vi "Integrator.vi"() -> ()   [LabVIEW 2019]
panel:
  out "Original Wave":dbl[](graph)=[0.0, 0.6180339887498948, 1.1755705045849463, 1.6180339887498947, 1.902113032590307, 2.0, 1.9021130325903073, 1.618033988749895, 1.1755705045849465, 0.6180339887498959, 2.4492935982947064e-16, -0.6180339887498946, -1.1755705045849454, -1.6180339887498936, -1.902113032590307, -2.0, -1.9021130325903073, -1.6180339887498962, -1.175570504584948, -0.6180339887498953, -4.898587196589413e-16, 0.6180339887498927, 1.1755705045849458, 1.6180339887498936, 1.9021130325903064, 2.0, 1.9021130325903084, 1.6180339887498951, 1.1755705045849467, 0.6180339887498989, 7.347880794884119e-16, -0.6180339887498908, -1.1755705045849456, -1.6180339887498945, -1.9021130325903057, -2.0, -1.9021130325903086, -1.6180339887498953, -1.175570504584947, -0.6180339887498991]
  in  "Amplitude":dbl=2.0
  out "Integrated Wave":dbl[](graph)=[0.0, 6.180339887498948e-05, 0.0001793604493334841, 0.0003411638482084736, 0.0005313751514675043, 0.0007313751514675043, 0.000921586454726535, 0.0010833898536015245, 0.0012009469040600192, 0.0012627503029350087, 0.0012627503029350087, 0.0012009469040600192, 0.0010833898536015247, 0.0009215864547265354, 0.0007313751514675046, 0.0005313751514675046, 0.00034116384820847385, 0.00017936044933348423, 6.180339887498941e-05, -1.2197274440461925e-19, -1.7095861637051338e-19, 6.18033988749891e-05, 0.0001793604493334837, 0.0003411638482084731, 0.0005313751514675037, 0.0007313751514675037, 0.0009215864547265346, 0.001083389853601524, 0.0012009469040600187, 0.0012627503029350087, 0.0012627503029350087, 0.0012009469040600196, 0.001083389853601525, 0.0009215864547265357, 0.0007313751514675051, 0.0005313751514675052, 0.0003411638482084743, 0.00017936044933348474, 6.180339887499005e-05, 1.3552527156068805e-19]
  out "Integration Sum":dbl=1.3552527156068805e-19
  out "No. of\nsamples":dbl=40.0
  in  "No. of\ncycles":dbl=2.0
  in  "fs":dbl=10000.0
  in  "Phase":dbl
  in  "f":dbl=500.0
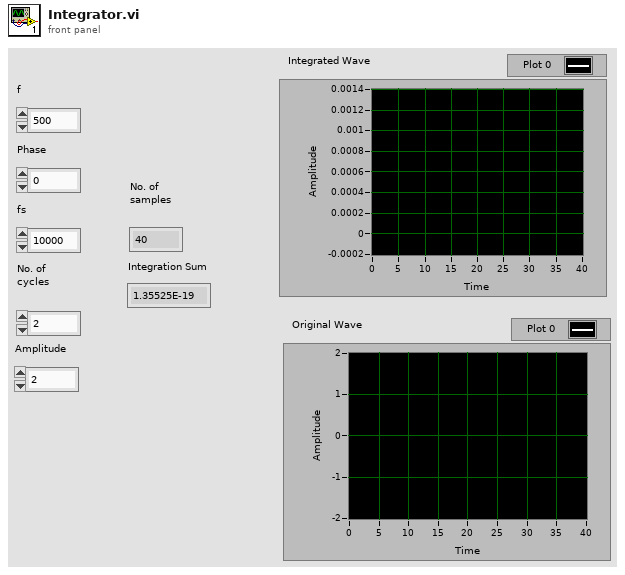
[diagram p1: front panel]
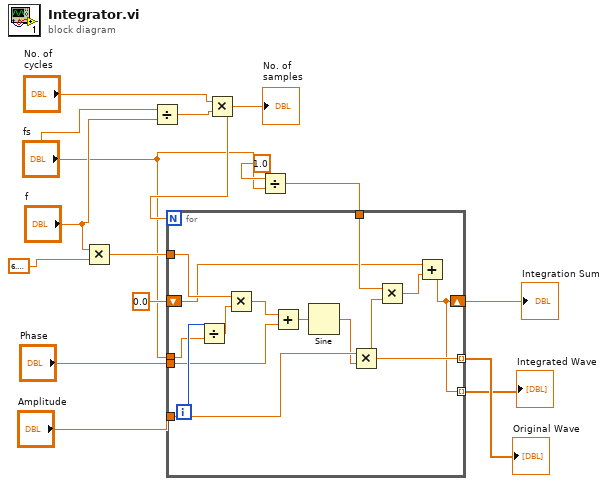
[diagram p0: block diagram]
diagram:
  n1 = Multiply(x="f", y=6.283185307179586) -> (x*y=w8:dbl)
  n2 = Divide(x="fs", y="f") -> (x/y=w15:dbl)
  n3 = Multiply(x="No. of\ncycles", y=w15) -> (x*y=w13:dbl)
  "No. of\nsamples" <- w13
  n4 = Divide(x=1.0, y="fs") -> (x/y=w6:dbl)
  n5 = for {
    N: w13 -> [_]
    tunnel: "fs" -> [w28]
    shift-right: [w16] -> w4
    shift-left: 0.0 ("x") -> [w17]
    tunnel: w8 -> [w26]
    tunnel: "Phase" -> [w24]
    tunnel: w6 -> [w23]
    tunnel: "Amplitude" -> [w22]
    tunnel: [w19] -> w2 mode=indexing
    tunnel: [w16] -> w1 mode=indexing
    i -> [w29]
    n6 = Divide(x=w29, y=w28) -> (x/y=w27:dbl)
    n7 = Multiply(x=w26, y=w27) -> (x*y=w25:dbl)
    n8 = Add(x=w25, y=w24) -> (x+y=w21:dbl)
    n9 = Sine(x=w21) -> (sin(x)=w20:dbl)
    n10 = Multiply(x=w22, y=w20) -> (x*y=w19:dbl)
    n11 = Multiply(x=w23, y=w19) -> (x*y=w18:dbl)
    n12 = Add(x=w17, y=w18) -> (x+y=w16:dbl)
  }
  "Integration Sum" <- w4
  "Integrated Wave" <- w1
  "Original Wave" <- w2
